vi "Read Output.vi"(8 "error in (no error)":errorcluster, 11 "VISA resource name":refnum<visa-resource-name>) -> (0 "error out":errorcluster, 1 "Actual Current Level (A)":dbl format="%.2g", 2 "Actual Voltage Level (V)":dbl format="%.2g", 3 "VISA resource name out":refnum<visa-resource-name>)   [LabVIEW 2017, in "ScientiFic DC Power Supply.lvlib"]
doc: "Returns the actual voltage level and actual current level for a desired channel."
uses:
  ScientiFic DC Power Supply.lvlib
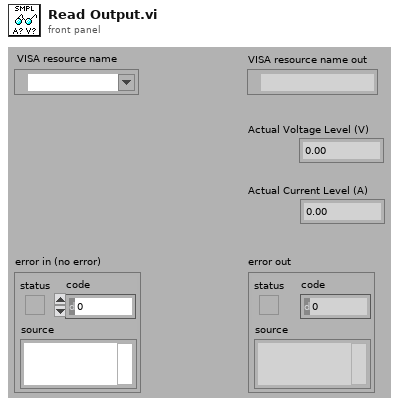
[diagram p1: front panel]
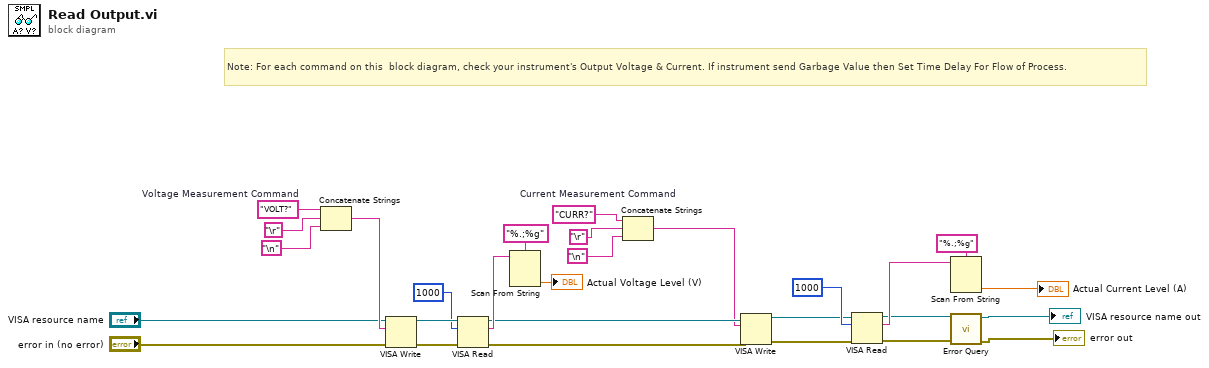
[diagram p0: block diagram]
diagram:
  w4 = "CURR?"  # Current Measurement Command
  w8 = "VOLT?"  # Voltage Measurement Command
  # "Note: For each command on this  block diagram, check your instrument's Output Voltage & Current. If instrument send Garbage Value then Set Time Delay For Flow of Process."
  n1 = Concatenate Strings(w8, "\r", "\n") -> (w7:string)
  n2 = VISA Write(VISA resource name="VISA resource name", write buffer=w7, error in (no error)="error in (no error)") -> (VISA resource name out=w27:refnum<visa-resource-name>, error out=w28:errorcluster)  [unwired: 1 out]
  n3 = VISA Read(VISA resource name=w27, byte count=u32 1000, error in (no error)=w28) -> (VISA resource name out=w11:refnum<visa-resource-name>, read buffer=w22:string, error out=w12:errorcluster)  [unwired: 1 out]
  n4 = Scan From String(format string="%.;%g", input string=w22) -> (output 1=→"Actual Voltage Level (V)":dbl)  [unwired: 3 in, 3 out]
  n5 = Concatenate Strings(w4, "\r", "\n") -> (w3:string)
  n6 = VISA Write(VISA resource name=w11, write buffer=w3, error in (no error)=w12) -> (VISA resource name out=w17:refnum<visa-resource-name>, error out=w16:errorcluster)  [unwired: 1 out]
  n7 = VISA Read(VISA resource name=w17, byte count=u32 1000, error in (no error)=w16) -> (VISA resource name out=w14:refnum<visa-resource-name>, read buffer=w19:string, error out=w13:errorcluster)  [unwired: 1 out]
  n8 = Scan From String(format string="%.;%g", input string=w19) -> (output 1=→"Actual Current Level (A)":dbl)  [unwired: 3 in, 3 out]
  n9 = call "Error Query.vi"("error in (no error)"=w13, "VISA resource name"=w14) -> ("error out"=→"error out":errorcluster, "VISA resource name out"=→"VISA resource name out":refnum<visa-resource-name>)  [unwired: 8 in]
